vi "DI_init.vi"(4 "DIParamTable":string="fd_3", 5 "KFM":string[](array[string]), 6 "conninfo":T1={"host"="localhost", "port"="5432", "client_encoding"="WIN1251", "dbname"="data", "user"="postgres", "password"=""}, 7 "N_param":i32, 9 "Names def":string[][](array[string]), 10 "Parameters def":dbl[][](array[numeric]), 11 "DIParameters":string[](array[string])) -> (0 "error":errorcluster, 3 "DI out":T2)   [LabVIEW 2019, in "Inputs.lvlib"]
uses:
  Inputs.lvlib
  Ctl/DI.ctl
  Ctl/DI short.ctl
  Ctl/Parameter State.ctl
  Database/ctl/Coninfo.ctl
  Database/PostgreSQL.lvlib
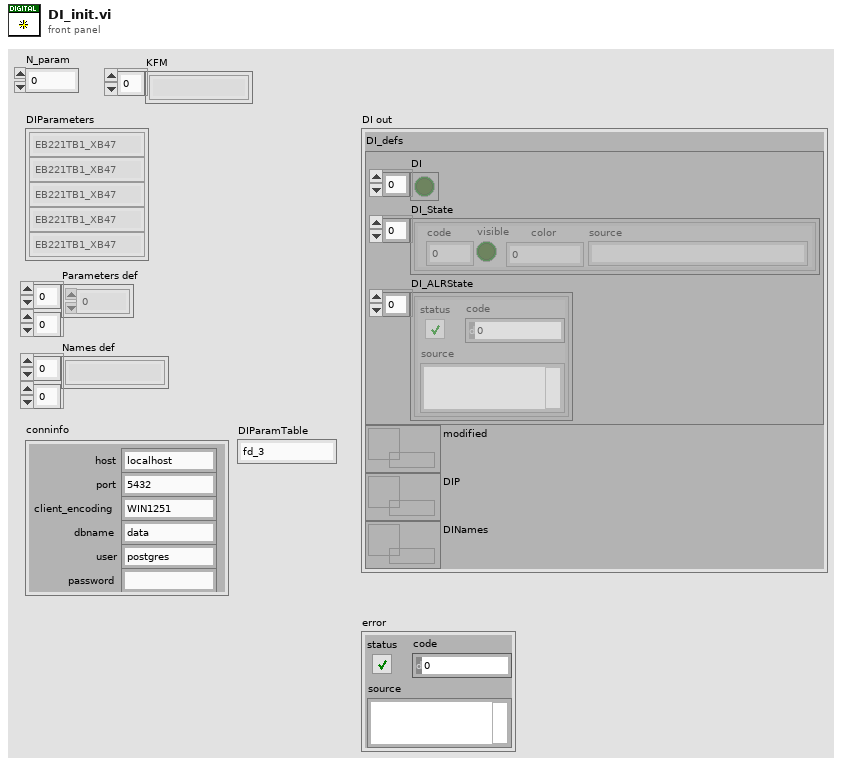
[diagram p1: front panel]
types:
  T1 = typedef "PostgreSQL.lvlib/Coninfo.ctl" = cluster{"host":string, "port":string, "client_encoding":string, "dbname":string, "user":string, "password":string}
  T2 = typedef "Inputs.lvlib/DI.ctl" = cluster{"DI_defs":T3, "modified":refnum<data-value>, "DIP":refnum<data-value>, "DINames":refnum<data-value>}
  T3 = typedef "Inputs.lvlib/DI short.ctl" = cluster{"DI":bool[], "DI_State":T4[], "DI_ALRState":errorcluster[]}
  T4 = typedef "Inputs.lvlib/Parameter State.ctl" = cluster{"code":i32, "visible":bool, "color":u32, "source":string}
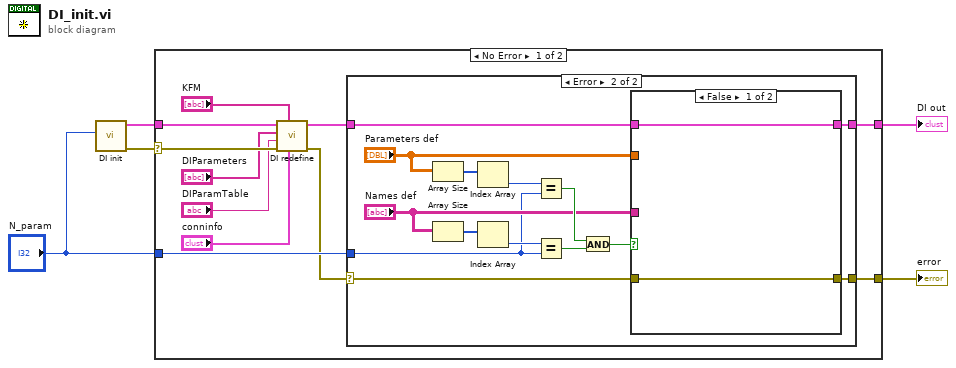
[diagram p0: block diagram]
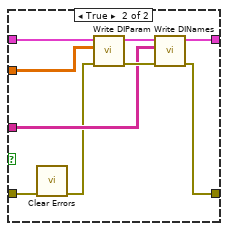
[diagram p3: hidden frame]
diagram:
  n1 = call "DI init.vi"("N_param"="N_param") -> ("error"=w2:errorcluster, "DI"=w3:T2)  [unwired: 9 in]
  n2 = case shown="No Error" w2 {
    selector: w2 -> [w13 w45]
    tunnel: "N_param" -> [w15 _]
    tunnel: [w16 w45] -> w5
    tunnel: w3 -> [w12 w44]
    tunnel: [w14 w44] -> w1
    frame No Error {
      n3 = call "DI redefine.vi"("conninfo"="conninfo", "KFM"="KFM", "error in (no error)"=w13, "DIParamTable"="DIParamTable", "DIParameters"="DIParameters", "DI in"=w12) -> ("error"=w10:errorcluster, "DI out"=w11:T2)  [unwired: 4 in]
      n4 = case shown="Error" w10 {
        selector: w10 -> [w18 w23]
        tunnel: [w18 w24] -> w16
        tunnel: w15 -> [_ w25]
        tunnel: w11 -> [w17 w20]
        tunnel: [w17 w19] -> w14
        frame No Error {
        }
        frame Error {
          n5 = Array Size(array="Parameters def") -> (size(s)=w27:i32[])
          n6 = Array Size(array="Names def") -> (size(s)=w28:i32[])
          n7 = Index Array(array=w27) -> (element=w29:i32)  [unwired: 1 in]
          n8 = Index Array(array=w28) -> (element=w30:i32)  [unwired: 1 in]
          n9 = Equal?(x=w29, y=w25) -> (x = y?=w31:bool)
          n10 = Equal?(x=w30, y=w25) -> (x = y?=w32:bool)
          n11 = And(x=w31, y=w32) -> (x .and. y?=w21:bool)
          n12 = case shown="False" w21 {
            tunnel: "Parameters def" -> [_ w37]
            tunnel: "Names def" -> [_ w38]
            tunnel: [w33 w39] -> w24
            tunnel: w23 -> [w33 w36]
            tunnel: w20 -> [w34 w41]
            tunnel: [w34 w40] -> w19
            frame False {
            }
            frame True {
              n13 = call <vilib>:"Clear Errors.vi"("error in (no error)"=w36) -> ("error out"=w35:errorcluster)  [unwired: 5 in, 1 out]
              n14 = call "Write DIParam.vi"("error in (no error)"=w35, "DIParam"=w37, "DI in"=w41) -> ("error out"=w42:errorcluster, "DI out"=w43:T2)  [unwired: 7 in]
              n15 = call "Write DINames.vi"("error in (no error)"=w42, "DINames"=w38, "DI in"=w43) -> ("error out"=w39:errorcluster, "DI out"=w40:T2)  [unwired: 7 in]
            }
          }
        }
      }
    }
    frame Error {
    }
  }
  "DI out" <- w1
  "error" <- w5
